vi "DCVM Analyze DC Voltage Measurements.vi"(0 "Voltage Waveforms":waveform(dbl)[](array[waveform]), 11 "error in (no error)":errorcluster) -> (4 "DC and RMS Voltage Measurements":T1 {"RMS Voltage (V)" format="%.2p"; "Average DC Voltage (V)" format="%.2p"}, 15 "error out":errorcluster)   [LabVIEW 2021, in "DAQ_DC-RMS Voltage Measurement.lvlib"]
doc: "Analyzes the DC voltage waveform data to derive required DC-RMS Voltage measurements"
uses:
  DAQ_DC-RMS Voltage Measurement.lvlib
  Typedefs/DC and RMS Voltage Measurements.ctl
  <vilib>/measure/madcrms.llb/Basic Averaged DC-RMS for N Chan.vi
  <vilib>/measure/NI_MAPro.lvlib
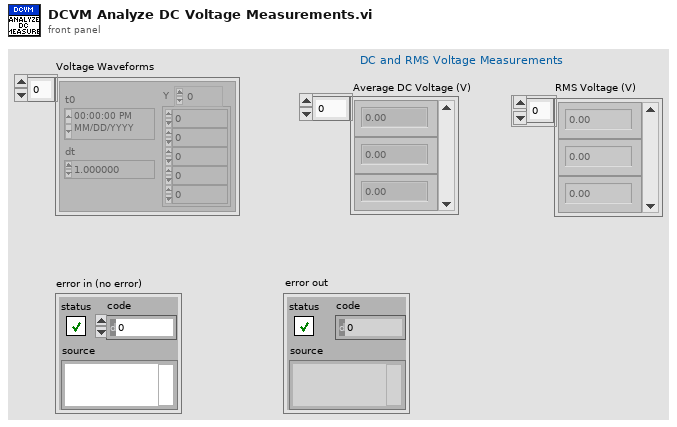
[diagram p1: front panel]
types:
  T1 = typedef "DAQ_DC-RMS Voltage Measurement.lvlib/DC and RMS Voltage Measurements.ctl" = cluster{"Average DC Voltage (V)":dbl[], "RMS Voltage (V)":dbl[]}
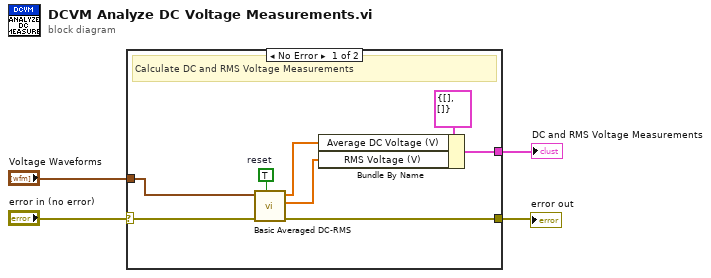
[diagram p0: block diagram]
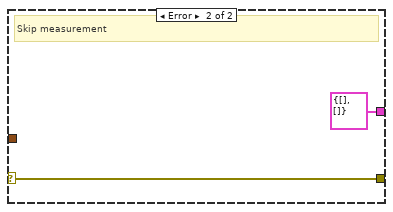
[diagram p2: hidden frame]
diagram:
  n1 = case shown="No Error" "error in (no error)" {
    selector: "error in (no error)" -> [w12 w13]
    tunnel: [w11 w13] -> w3
    tunnel: "Voltage Waveforms" -> [w10 _]
    tunnel: [w8 T1 {"Average DC Voltage (V)"=[], "RMS Voltage (V)"=[]} ("DC Measurements")] -> w1
    frame No Error {
      w5 = TRUE  # reset
      # "Calculate DC and RMS Voltage Measurements"
      n2 = call-poly <vilib>:"Basic Averaged DC-RMS.vi"("reset"=w5, "error in (no error)"=w12, "signals in"=w10) -> ("error out"=w11:errorcluster, "RMS values"=w6:dbl[], "DC values"=w7:dbl[])  [unwired: 5 in, 1 out]
      n3 = Bundle By Name(cluster=T1 {"Average DC Voltage (V)"=[], "RMS Voltage (V)"=[]} ("DC Measurements"), "Average DC Voltage (V)"=w7, "RMS Voltage (V)"=w6) -> (w8:T1)
    }
    frame Error {
      # "Skip measurement"
    }
  }
  "error out" <- w3
  "DC and RMS Voltage Measurements" <- w1
